vi "Defined Channel Range Specifier.vi"(8 "error in":errorcluster, 10 "Card":T2(ring), 11 "Buffer":T1(ring)) -> (0 "error out":errorcluster, 3 "Channel Range":string)   [LabVIEW 2018]
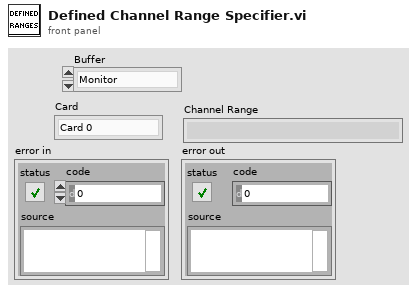
[diagram p1: front panel]
types:
  T1 = enum16{"Monitor", "Demand", "Backup", "All", "None"}
  T2 = enum16{"Card 0", "Card 1", "Card 2", "Card 3", "Card 4", "Card 5", "Card 6", "Card 7", "Card 8", "Card 9", "Card 10", "Card 11", "Card 12", "Card 13", "Card 14", "Card 15"}
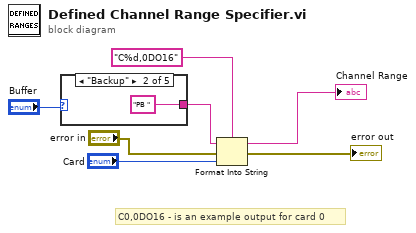
[diagram p0: block diagram]
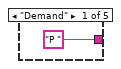
[diagram p2: hidden frame]
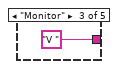
[diagram p3: hidden frame]
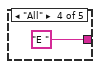
[diagram p4: hidden frame]
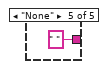
[diagram p5: hidden frame]
diagram:
  # "C0,0DO16 - is an example output for card 0"
  n1 = case shown="\"Backup\"" "Buffer" {
    tunnel: ["P " "PB " "V " "E " " "] -> w2
    frame "Demand" {
    }
    frame "Backup" {
    }
    frame "Monitor" {
    }
    frame "All" {
    }
    frame "None" {
    }
  }
  n2 = Format Into String(format string="C%d,0DO16", initial string=w2, error in="error in", "Card") -> (resulting string=→"Channel Range":string, error out=→"error out":errorcluster)
